vi "FL_Calculate_Coordinates.vi"(0 "Input cluster":cluster{"X1":dbl, "Y1":dbl, "X2":dbl, "Y2":dbl}) -> (9 "X1-X2":sgl, 11 "Y1-Y2":sgl, 14 "sin(a)":sgl, 15 "R from center":sgl, 16 "Mouse Xc":sgl, 17 "Mouse Yc":sgl, 18 "Cage Xc":sgl, 19 "Cage Yc":sgl)   [LabVIEW 2018]
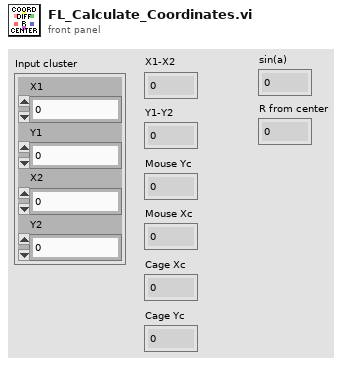
[diagram p1: front panel]
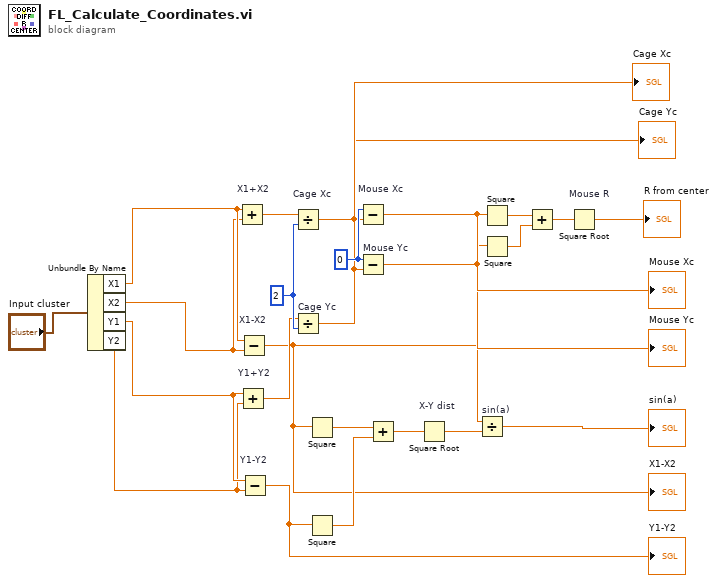
[diagram p0: block diagram]
diagram:
  w14 = 0
  w17 = 2
  n1 = Unbundle By Name("Input cluster") -> ("X1"=w4:dbl, "X2"=w3:dbl, "Y1"=w2:dbl, "Y2"=w1:dbl)
  n2 = Add "X1+X2"(x=w4, y=w3) -> (x+y=w15:dbl)
  n3 = Add "Y1+Y2"(x=w2, y=w1) -> (x+y=w16:dbl)
  n4 = Subtract "X1-X2"(x=w4, y=w3) -> (x-y=w7:dbl)
  "X1-X2" <- w7
  n5 = Subtract "Y1-Y2"(x=w2, y=w1) -> (x-y=w8:dbl)
  "Y1-Y2" <- w8
  n6 = Divide "Cage Xc"(x=w15, y=w17) -> (x/y=w13:dbl)
  "Cage Xc" <- w13
  n7 = Divide "Cage Yc"(x=w16, y=w17) -> (x/y=w12:dbl)
  "Cage Yc" <- w12
  n8 = Square(x=w7) -> (x^2=w18:dbl)
  n9 = Square(x=w8) -> (x^2=w19:dbl)
  n10 = Subtract "Mouse Xc"(x=w14, y=w13) -> (x-y=w11:dbl)
  "Mouse Xc" <- w11
  n11 = Subtract "Mouse Yc"(x=w14, y=w12) -> (x-y=w10:dbl)
  "Mouse Yc" <- w10
  n12 = Add(x=w18, y=w19) -> (x+y=w20:dbl)
  n13 = Square Root "X-Y dist"(x=w20) -> (sqrt(x)=w21:dbl)
  n14 = Divide "sin(a)"(x=w7, y=w21) -> (x/y=→"sin(a)":dbl)
  n15 = Square(x=w11) -> (x^2=w22:dbl)
  n16 = Square(x=w10) -> (x^2=w23:dbl)
  n17 = Add(x=w22, y=w23) -> (x+y=w24:dbl)
  n18 = Square Root "Mouse R"(x=w24) -> (sqrt(x)=→"R from center":dbl)
